vi "HRTF-Copy Speaker Only Data.vi"(0 "to":path, 5 "from":path) -> (15 "error out":errorcluster)   [LabVIEW 2015]
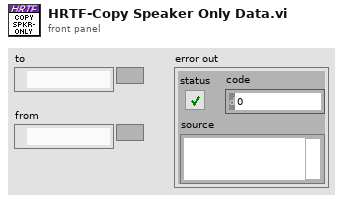
[diagram p1: front panel]
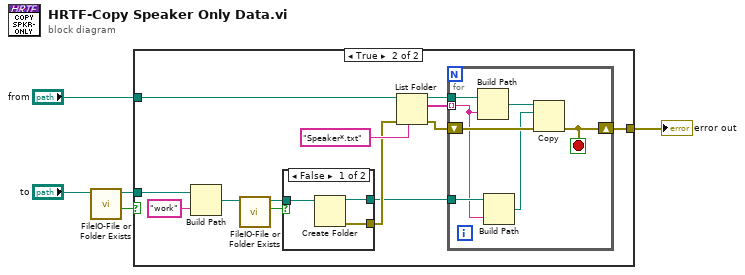
[diagram p0: block diagram]
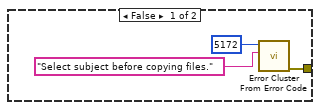
[diagram p2: hidden frame]
diagram:
  n1 = call "FileIO-File or Folder Exists.vi"("path"="to") -> ("Exists?"=w4:bool, "dup path"=w3:path)  [unwired: 7 in, 2 out]
  n2 = case shown="True" w4 {
    tunnel: w3 -> [_ w21]
    tunnel: "from" -> [_ w16]
    tunnel: [w8 w9] -> w1
    frame False {
      n3 = call <vilib>:"Error Cluster From Error Code.vi"("error message (\"\")"="Select subject before copying files." ("error message (\"\")"), "error code (0)"=5172) -> ("error out"=w8:errorcluster)  [unwired: 7 in]
    }
    frame True {
      n4 = Build Path(base path=w21, name or relative path="work") -> (appended path=w19:path)
      n5 = call "FileIO-File or Folder Exists.vi"("path"=w19) -> ("Directory?"=w18:bool, "dup path"=w17:path)  [unwired: 7 in, 2 out]
      n6 = case shown="False" w18 {
        tunnel: w17 -> [w31 w32]
        tunnel: [w30 w32] -> w10
        tunnel: [w29 _] -> w13
        frame False {
          n7 = Create Folder(path (use dialog)=w31) -> (created path=w30:path, error out=w29:errorcluster)  [unwired: 2 in, 1 out]
        }
        frame True {
        }
      }
      n8 = List Folder(path=w16, pattern="Speaker*.txt", error in=w13) -> (path out=w14:path, filenames=w12:string[], error out=w11:errorcluster)  [unwired: 1 in, 1 out]
      n9 = for {
        tunnel: w14 -> [w28]
        tunnel: w12 -> [w22] mode=indexing
        shift-right: [w25] -> w9
        shift-left: w11 -> [w26]
        tunnel: w10 -> [w24]
        stop <- w25 stop-if-true
        n10 = Build Path(base path=w28, name or relative path=w22) -> (appended path=w27:path)
        n11 = Build Path(base path=w24, name or relative path=w22) -> (appended path=w23:path)
        n12 = Copy(8:w26, 10:w23, 11:w27) -> (0:w25:errorcluster)  [unwired: 2 in, 2 out]
      }
    }
  }
  "error out" <- w1
